vi "Feature_Scorer.vi"(4 "Feature Scorer Params":T27={"Nearest_Neihbours"=1, "Calculate Anomaly Map"=TRUE, "Gaussian_Blur"={"Kernel_Size"=33, "sigma"=4.0}}, 8 "error in":errorcluster, 9 "bs, h, w, c1+..cN":i32[](array[numeric]), 10 "embedding":sgl[][](array[numeric]) format="%#_3p", 11 "PCore_Instance in":T1 {"NN out"."LR_Update_Policy"."WarmUp_Ratio" min=1; "NN out"."LR_Update_Policy"."WarmUp_Iter" min=1; "NN out"."LR_Update_Policy"."LR0" format="%.7f"; "Dataset_Stats"."vars"."R" format="%#_3g"; "Dataset_Stats"."vars"."G" format="%#_3g"; "Dataset_Stats"."vars"."B" format="%#_3g"; "Dataset_Stats"."means"."R" format="%#_3g"; "Dataset_Stats"."means"."G" format="%#_3g"; "Dataset_Stats"."means"."B" format="%#_3g"}) -> (0 "error out":errorcluster, 1 "anomaly map":sgl[][][](array[numeric]), 2 "pred score":sgl[](array[numeric]), 3 "PCore_Instance out":T1 {"NN out"."LR_Update_Policy"."WarmUp_Ratio" min=1; "NN out"."LR_Update_Policy"."WarmUp_Iter" min=1; "NN out"."LR_Update_Policy"."LR0" format="%.7f"; "Dataset_Stats"."vars"."R" format="%#_3g"; "Dataset_Stats"."vars"."G" format="%#_3g"; "Dataset_Stats"."vars"."B" format="%#_3g"; "Dataset_Stats"."means"."R" format="%#_3g"; "Dataset_Stats"."means"."G" format="%#_3g"; "Dataset_Stats"."means"."B" format="%#_3g"}, 5 "dT(pCore)":dbl)   [LabVIEW 2020]
uses:
  API/Controls/Feature_Scorer_Params.ctl
  API/Controls/Gaussian_Blur.ctl
  API/Controls/PatchCore_Instance.ctl
  API/Controls/PatchCore_DS_Stats.ctl
  API/Controls/Image_Stats_RGB.ctl
  <vilib>/Ngene/Deep Learning Toolkit/Toolkit/NN_Network/Controls/NN.ctl
  <vilib>/Ngene/Deep Learning Toolkit/Toolkit/NN_Layers/Controls/NN_Layer_ref.ctl
  <vilib>/Ngene/Deep Learning Toolkit/Toolkit/NN_Layers/Controls/NN_Layer.ctl
  <vilib>/Ngene/Deep Learning Toolkit/Toolkit/NN_Layers/Controls/NN_Layer_Type.ctl
  <vilib>/Ngene/Deep Learning Toolkit/Toolkit/NN_Data/API/NN_Dims(C,H,W).ctl
  <vilib>/Ngene/Deep Learning Toolkit/Toolkit/NN_Layers/Controls/NN_Layer_Metrics.ctl
  <vilib>/Ngene/Deep Learning Toolkit/Toolkit/NN_Network/Controls/NN_Device.ctl
  <vilib>/Ngene/Deep Learning Toolkit/Toolkit/NNg/cuda/Controls/nng_cuda_handles.ctl
  <vilib>/Ngene/Deep Learning Toolkit/Toolkit/NN_Layers/Controls/NN_Layer_Dimty.ctl
  <vilib>/Ngene/Deep Learning Toolkit/Toolkit/NN_Layers/Controls/NN_Layer_RF_State.ctl
  <vilib>/Ngene/Deep Learning Toolkit/Toolkit/NN_Data/API/NN_Dims(V,H).ctl
  <vilib>/Ngene/Deep Learning Toolkit/Toolkit/NN_Network/Controls/NN_In_Out_Dim-ty.ctl
  <vilib>/Ngene/Deep Learning Toolkit/Toolkit/NN_Train/Controls/NN_Train_Params.ctl
  <vilib>/Ngene/Deep Learning Toolkit/Toolkit/NN_Train/Controls/NN_Train_Optimizer.ctl
  <vilib>/Ngene/Deep Learning Toolkit/Toolkit/NN_Train/Controls/NN_Train_Data_Sampling.ctl
  <vilib>/Ngene/Deep Learning Toolkit/Toolkit/NN_Train/Controls/NN_LR_Policy_Cfg.ctl
  <vilib>/Ngene/Deep Learning Toolkit/Toolkit/NN_Train/Controls/NN_LR_Policy_Type.ctl
  <vilib>/Ngene/Deep Learning Toolkit/Toolkit/NN_Train/Controls/NN_Train_Session_Data.ctl
  <vilib>/Ngene/Deep Learning Toolkit/Toolkit/NN_Data/Controls/NN_Ground_truth.ctl
  <vilib>/Ngene/Deep Learning Toolkit/Toolkit/NN_Train/Controls/NN_Loss_Type.ctl
  <vilib>/Ngene/Deep Learning Toolkit/Toolkit/NNg/Network/WS/Controls/NNG_WS.ctl
  <vilib>/Ngene/Deep Learning Toolkit/Toolkit/NNg/Network/WS/Controls/NNg_WS_Mem_DVR.ctl
  <vilib>/Ngene/Deep Learning Toolkit/Toolkit/NNg/cuda/Controls/cuda_Mem_desc.ctl
  API/Controls/PCore_Device.ctl
  API/Controls/PatchCore_Init_CFG.ctl
  API/Controls/PatchCore_BackBone_Selector.ctl
  API/Controls/Coreset_Params.ctl
  API/Controls/Random_Projection_Coreset.ctl
  API/Controls/MemBank_and_Norm_Variants.ctl
  <vilib>/Ngene/Deep Learning Toolkit/Toolkit/NN_Layers/Layers/Input/subVIs/Augmentation/Blur/Gauss_Blur.vi
  Interpolate_Align_Corners=False.vi
  <vilib>/Ngene/Deep Learning Toolkit/Toolkit/NN_Layers/Layers/Input/subVIs/Augmentation/Blur/SubVI/Gauss_Function.vi
  <vilib>/Utility/High Resolution Relative Seconds.vi
  Intrplt_Get_Dest_Coords.vi
  <vilib>/addons/Multicore Analysis and Sparse Matrix/Signal Operation/Convolution.vi
  <vilib>/addons/Multicore Analysis and Sparse Matrix/Signal Operation/_sigop/2D Convolution (SGL).vi
  <vilib>/Ngene/Deep Learning Toolkit/Toolkit/Deep_Learning_Toolkit_by_Ngene.lvlib
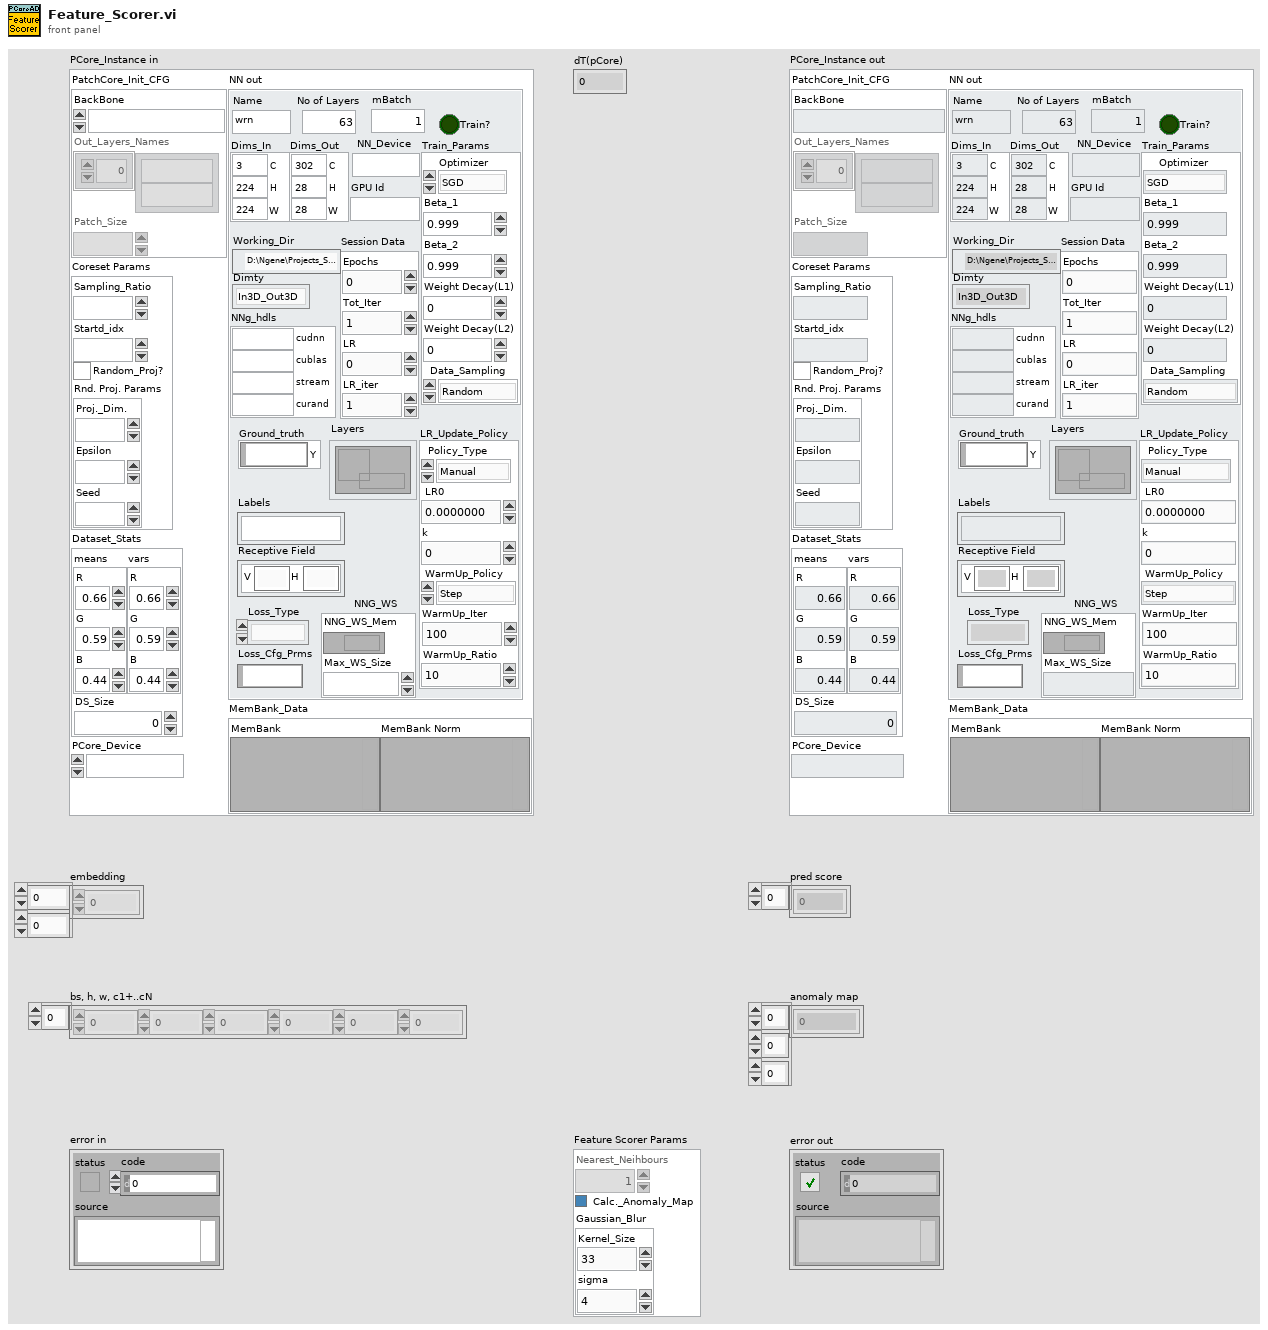
[diagram p1: front panel]
types:
  T1 = typedef "PatchCore_Instance.ctl" = cluster{"Dataset_Stats":T2, "NN":T4, "PCore_Device":T21, "PatchCore_Init_CFG":T22, "Coreset Params":T24, "MemBank_Data":T26}
  T2 = typedef "PatchCore_DS_Stats.ctl" = cluster{"means":T3, "vars":T3, "DS_Size":i32}
  T3 = typedef "Image_Stats_RGB.ctl" = cluster{"R":sgl, "G":sgl, "B":sgl}
  T4 = typedef "Deep_Learning_Toolkit_by_Ngene.lvlib/NN.ctl" = cluster{"Name":string, "No of Layers":i32, "mBatch":i32, "Layers":T5[], "Dimty":T6, "Dims_In":T7, "Dims_Out":T7, "Working_Dir":path, "Train?":bool, "Train_Params":T8, "LR_Update_Policy":T11, "Session Data":T13, "Ground_truth":T14, "NNg_hdls":T15, "NN_Device":T16, "GPU Id":i32, "Labels":string[], "Receptive Field":T17[], "Loss_Type":T18, "Loss_Cfg_Prms":variant, "NNG_WS":T19}
  T5 = typedef "Deep_Learning_Toolkit_by_Ngene.lvlib/NN_Layer_ref.ctl" = refnum<data-value>
  T6 = typedef "Deep_Learning_Toolkit_by_Ngene.lvlib/NN_In_Out_Dim-ty.ctl" = enum8{"In1D_Out1D", "In3D_Out1D", "In3D_Out3D", "In3D_OutBBox"}
  T7 = typedef "Deep_Learning_Toolkit_by_Ngene.lvlib/NN_Dims(C,H,W).ctl" = cluster{"C":i32, "H":i32, "W":i32}
  T8 = typedef "Deep_Learning_Toolkit_by_Ngene.lvlib/NN_Train_Params.ctl" = cluster{"Optimizer":T9, "Beta_1":sgl, "Beta_2":sgl, "Weight Decay(L1)":sgl, "Weight Decay(L2)":sgl, "Data_Sampling":T10}
  T9 = typedef "Deep_Learning_Toolkit_by_Ngene.lvlib/NN_Train_Optimizer.ctl" = enum16{"SGD", "Adam", "Adagrad", "Adadelta", "RMSProp", "Nesterov"}
  T10 = typedef "Deep_Learning_Toolkit_by_Ngene.lvlib/NN_Train_Data_Sampling.ctl" = enum16{"Random", "Sequential"}
  T11 = typedef "Deep_Learning_Toolkit_by_Ngene.lvlib/NN_LR_Policy_Cfg.ctl" = cluster{"Policy_Type":T12, "LR0":dbl, "k":sgl, "WarmUp_Policy":enum16{"Step", "Ramp"}, "WarmUp_Iter":i32, "WarmUp_Ratio":sgl}
  T12 = typedef "Deep_Learning_Toolkit_by_Ngene.lvlib/NN_LR_Policy_Type.ctl" = enum16{"Manual", "Step", "Exp", "1/t"}
  T13 = typedef "Deep_Learning_Toolkit_by_Ngene.lvlib/NN_Train_Session_Data.ctl" = cluster{"Epochs":sgl, "Tot_Iter":i32, "LR":sgl, "LR_iter":i32}
  T14 = typedef "Deep_Learning_Toolkit_by_Ngene.lvlib/NN_Ground_truth.ctl" = cluster{"Y":variant}
  T15 = typedef "Deep_Learning_Toolkit_by_Ngene.lvlib/nng_cuda_handles.ctl" = cluster{"cudnn":u64, "cublas":u64, "stream":u64, "curand":u64}
  T16 = typedef "Deep_Learning_Toolkit_by_Ngene.lvlib/NN_Device.ctl" = enum16{"CPU", "GPU"}
  T17 = typedef "Deep_Learning_Toolkit_by_Ngene.lvlib/NN_Dims(V,H).ctl" = cluster{"V":i32, "H":i32}
  T18 = typedef "Deep_Learning_Toolkit_by_Ngene.lvlib/NN_Loss_Type.ctl" = enum16{"None", "MSE", "CrossEntropy", "YOLO_v2", "YOLO_v4"}
  T19 = typedef "Deep_Learning_Toolkit_by_Ngene.lvlib/NNG_WS.ctl" = cluster{"NNG_WS_Mem":T20, "Max_WS_Size":i64}
  T20 = typedef "Deep_Learning_Toolkit_by_Ngene.lvlib/NNg_WS_Mem_DVR.ctl" = refnum<data-value>
  T21 = typedef "PCore_Device.ctl" = enum16{"CPU", "GPU(CuLab)"}
  T22 = typedef "PatchCore_Init_CFG.ctl" = cluster{"BackBone":T23, "Out_Layers_Names":string[], "Patch_Size":u32}
  T23 = typedef "PatchCore_BackBone_Selector.ctl" = enum16{"WRN_50_2_L2L3"}
  T24 = typedef "Coreset_Params.ctl" = cluster{"Sampling_Ratio":sgl, "Startd_idx":i32, "Random_Proj?":bool, "Rnd. Proj. Params":T25}
  T25 = typedef "Random_Projection_Coreset.ctl" = cluster{"Proj._Dim.":i32, "Epsilon":sgl, "Seed":i32}
  T26 = typedef "MemBank_and_Norm_Variants.ctl" = cluster{"MemBank":variant, "MemBank Norm":variant}
  T27 = typedef "Feature_Scorer_Params.ctl" = cluster{"Nearest_Neihbours":i32, "Calculate Anomaly Map":bool, "Gaussian_Blur":T28}
  T28 = typedef "Gaussian_Blur.ctl" = cluster{"Kernel_Size":i32, "sigma":sgl}
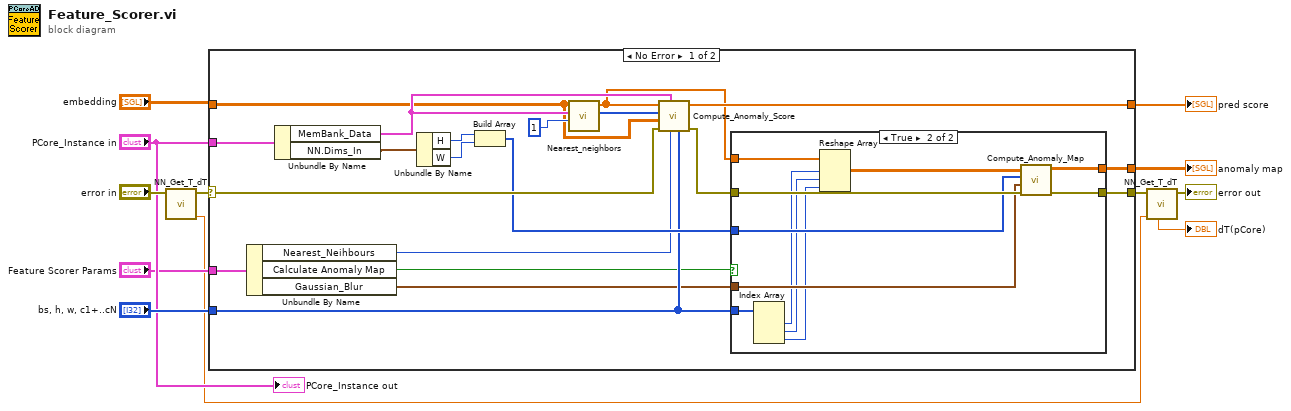
[diagram p0: block diagram]
diagram:
  n1 = call <vilib>:"NN_Get_T_dT.vi"("error in (no error)"="error in") -> ("T_out"=w1:dbl, "error out"=w4:errorcluster)  [unwired: 6 in, 1 out]
  n2 = case shown="No Error" w4 {
    selector: w4 -> [w31 w45]
    tunnel: "bs, h, w, c1+..cN" -> [w23 _]
    tunnel: "embedding" -> [w15 _]
    tunnel: [w14 _] -> w8
    tunnel: [w32 _] -> w11
    tunnel: [w30 w45] -> w9
    tunnel: "PCore_Instance in" -> [w22 _]
    tunnel: "Feature Scorer Params" -> [w21 _]
    frame No Error {
      n3 = Unbundle By Name(w21) -> ("Nearest_Neihbours"=w17:i32, "Calculate Anomaly Map"=w20:bool, "Gaussian_Blur"=w19:T28)
      n4 = Unbundle By Name(w22) -> ("MemBank_Data"=w16:T26, "NN.Dims_In"=w18:T7)
      n5 = Unbundle By Name(w18) -> ("H"=w28:i32, "W"=w27:i32)
      n6 = Build Array(w28, w27) -> (w26:i32[])
      n7 = call "Nearest_neighbors.vi"("n neighbors"=1, "Membank"=w16, "Features"=w15) -> ("locations"=w24:i32[], "patch scores"=w13:sgl[])  [unwired: 4 in, 3 out]
      n8 = call "Compute_Anomaly_Score.vi"("bs, h, w, c1+..cN"=w23, "n neighbors"=w17, "Membank"=w16, "error in"=w31, "embedding"=w15, "locations"=w24, "patch scores"=w13) -> ("error out"=w29:errorcluster, "image-lvl anomaly score"=w14:sgl[])  [unwired: 3 in]
      n9 = case shown="True" w20 {
        tunnel: [_ w34] -> w32
        tunnel: [w33 w44] -> w30
        tunnel: w29 -> [w33 w43]
        tunnel: w19 -> [_ w42]
        tunnel: w26 -> [_ w41]
        tunnel: w13 -> [_ w39]
        tunnel: w23 -> [_ w38]
        frame False {
        }
        frame True {
          n10 = Index Array(array=w38) -> (element #1=w37:i32, element #2=w36:i32, element #3=w35:i32)  [unwired: 3 in]
          n11 = Reshape Array(w39, w37, w36, w35) -> (w40:sgl[][][])
          n12 = call "Compute_Anomaly_Map.vi"("error in"=w43, "Gaussian Blur"=w42, "input img size"=w41, "patch scores [bs,h,w]"=w40) -> ("error IO"=w44:errorcluster, "anomaly map"=w34:sgl[][][])  [unwired: 6 in]
        }
      }
    }
    frame Error {
    }
  }
  "pred score" <- w8
  "anomaly map" <- w11
  n13 = call <vilib>:"NN_Get_T_dT.vi"("T_in"=w1, "error in (no error)"=w9) -> ("error out"=→"error out":errorcluster, "dT"=→"dT(pCore)":dbl)  [unwired: 5 in, 1 out]
  "PCore_Instance out" <- "PCore_Instance in"
